vi "欣然动力数据采集系统.vi"() -> ()   [LabVIEW 2020]
uses:
  <vilib>/Utility/error.llb/DialogType.ctl
  <userlib>/ArtDAQ/_SubVI/ArtDAQ_CreateAIVoltageChan.vi
  <userlib>/ArtDAQ/_SubVI/ArtDAQ_CfgSampClkTiming.vi
  <userlib>/ArtDAQ/_SubVI/ArtDAQ_Read Analog DBL NChan NSamp.vi
  <vilib>/express/express analysis/Spectral/Block/exnSpectralBlock spectral measurements RMS poly.vi
  <vilib>/express/express analysis/Spectral/Block/exnSpectralBlock spectral measurements RMS WFM.vi
  <userlib>/ArtDAQ/_SubVI/ArtDAQ_CreateCIFreqChan.vi
  <userlib>/ArtDAQ/_SubVI/ArtDAQ_CfgImplicitTiming.vi
  <userlib>/ArtDAQ/_SubVI/ArtDAQ_Read Counter DBL NSamp.vi
  <vilib>/express/express analysis/Spectral/XNode/ExpressSpectralMeasurementsBlockNode.xnode
panel:
  out "排温2raw":dbl
  out "排温1raw":dbl format="%#.1f"
  out "推力raw":dbl caption="推力" format="%#.1f"
  in  "?":enum32{"通道及记录设置", "参数显示", "振动显示"}(tab)
  in  "流量通道":string="Dev1/ctr1"
  in  "震动通道3":string="Dev1/ai3"
  in  "震动通道2":string="Dev1/ai2"
  in  "震动通道1":string="Dev1/ai1"
  in  "排温通道2":string="Dev1/ai13"
  in  "排温通道1":string="Dev1/ai9"
  in  "推力通道":string="Dev1/ai0"
  in  "大气温度通道":string="Dev1/ai12"
  in  "大气压力通道":string="Dev1/ai11"
  in  "Filename":path=path "vibration.tdms" caption="振动参数"
  in  "记录频率":dbl=1.0
  in  "文件名":path=path "Engine_data.lvm" caption="发动机运行参数"
  in  "排温1超限报警值":dbl=800.0
  in  "排温2超限报警值":dbl=800.0
  in  "推力偏移校正":dbl
  in  "转速通道":string="Dev1/ctr0"
  in  "新建":bool
  in  "开始/暂停":bool
  out "?":dbl format="%#.0f"
  out "排温 2":dbl(knob) scale=0.0..1200.0
  out "?":dbl format="%#.0f"
  out "排温1":dbl(knob) scale=0.0..1200.0
  out "?":dbl format="%#.1f"
  out "推力":dbl(knob) scale=0.0..80.0
  out "?":dbl format="%#.1f"
  out "流量":dbl(knob) scale=0.0..3000.0
  out "?":dbl format="%#.0f"
  out "转速":dbl(knob) scale=0.0..100000.0 scale format="%#_3p"
  out "记录中 2":bool caption="记录中"
  out "发动机运行参数":dynamicdata(graph)=[{"t0"=timestamp(3721086911.630264 s since 1904-01-01), "dt"=0.1, "Y"=[0.0], "attributes"=variant("NI_ChannelName"=variant(string "滤波"))}, {"t0"=timestamp(3721086911.630264 s since 1904-01-01), "dt"=0.1, "Y"=[0.0], "attributes"=variant("NI_ChannelName"=variant(string "滤波"))}, {"t0"=timestamp(3721086911.630264 s since 1904-01-01), "dt"=0.1, "Y"=[-174.99999999999991], "attributes"=variant("NI_ChannelName"=variant(string "滤波"))}, {"t0"=timestamp(3721086911.630264 s since 1904-01-01), "dt"=0.1, "Y"=[0.0], "attributes"=variant("NI_ChannelName"=variant(string "滤波"))}, {"t0"=timestamp(3721086911.630264 s since 1904-01-01), "dt"=0.1, "Y"=[0.0], "attributes"=variant("NI_ChannelName"=variant(string "滤波"))}]
  out "大气压力":dbl format="%#.1f"
  out "机箱温度":dbl format="%#.1g"
  out "超温警报":bool
  in  "校零":bool
  in  "采样率":dbl=200000.0
  out "实际采样点数":dbl=30000.0
  in  "每循环采样数":i32=100000
  out "波形图 2":cluster{"f0":dbl, "df":dbl, "magnitude":dbl[]}(graph)
  in  "开始/暂停 2":bool
  in  "新建 2":bool
  out "波形图 3":cluster{"f0":dbl, "df":dbl, "magnitude":dbl[]}(graph) caption="波形图 2"
  out "波形图 4":cluster{"f0":dbl, "df":dbl, "magnitude":dbl[]}(graph) caption="波形图 2"
  out "加速度":waveform(dbl)[](graph)
  out "转速":dbl format="%#.0f"
  out "燃油流量":dbl caption="流量" format="%#.1f"
  # "参数记录设置"
  # "通道设置"
  # "记录频率"
  # "HZ"
  # "报警参数设置"
  # "参数校正"
  # "微型试车台数采系统 V1.1"
  # "欣然动力"
  # "kPa"
  # "r/min"
  # "ml/min"
  # "kgf"
  # "℃"
  # "℃"
  # "℃"
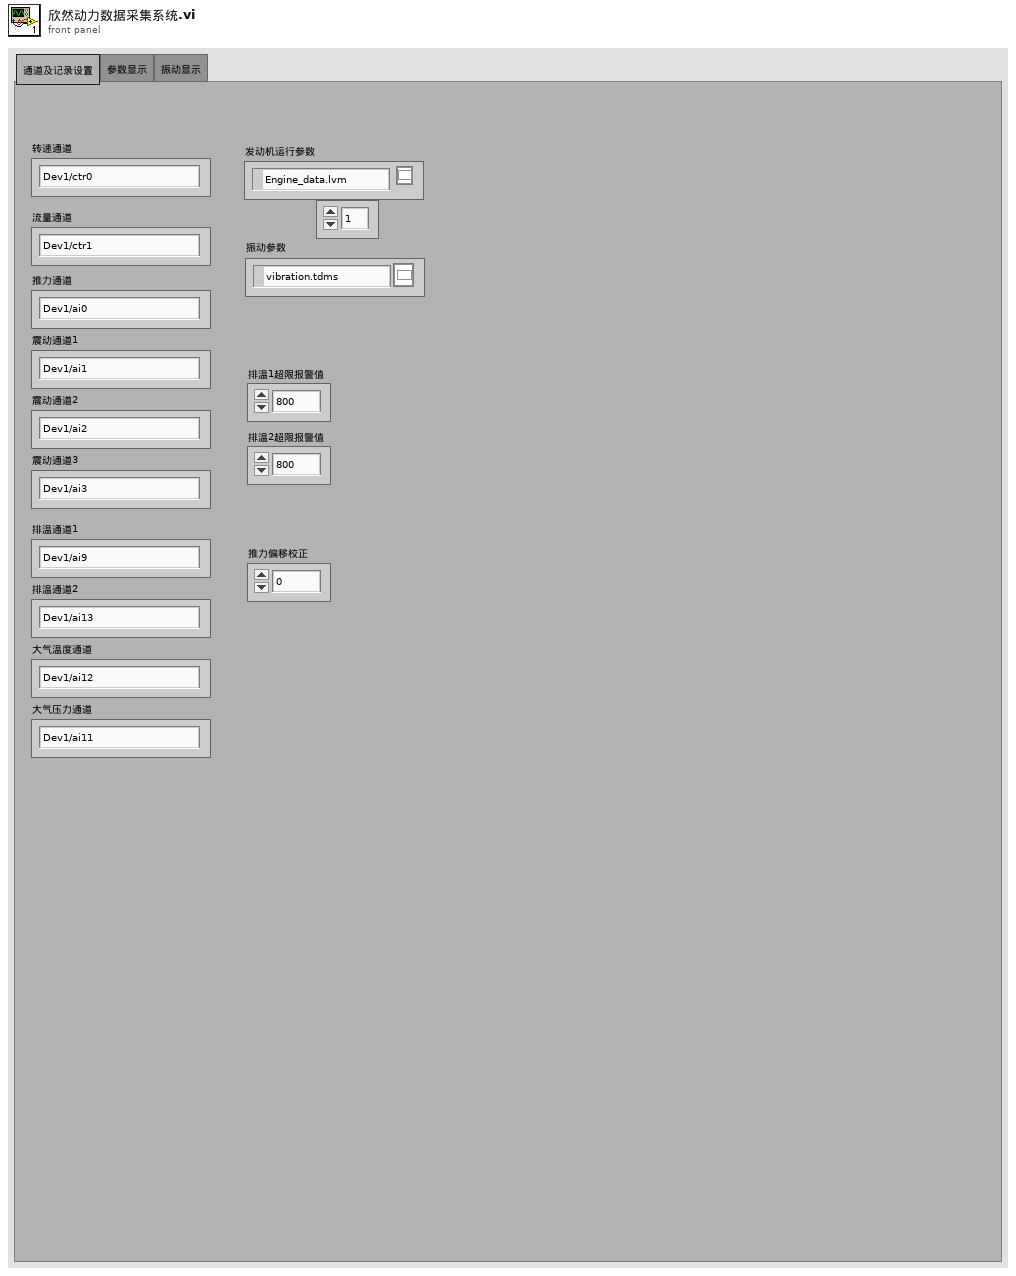
[diagram p1: front panel]
types:
  T1 = typedef "DialogType.ctl" = u16
  T2 = cluster{"averaging mode":u16, "weighting mode":u16, "number of averages":u32}
  T3 = cluster{"dB On (F)":bool, "unwrap phase (F)":bool, "convert to degree (F)":bool}
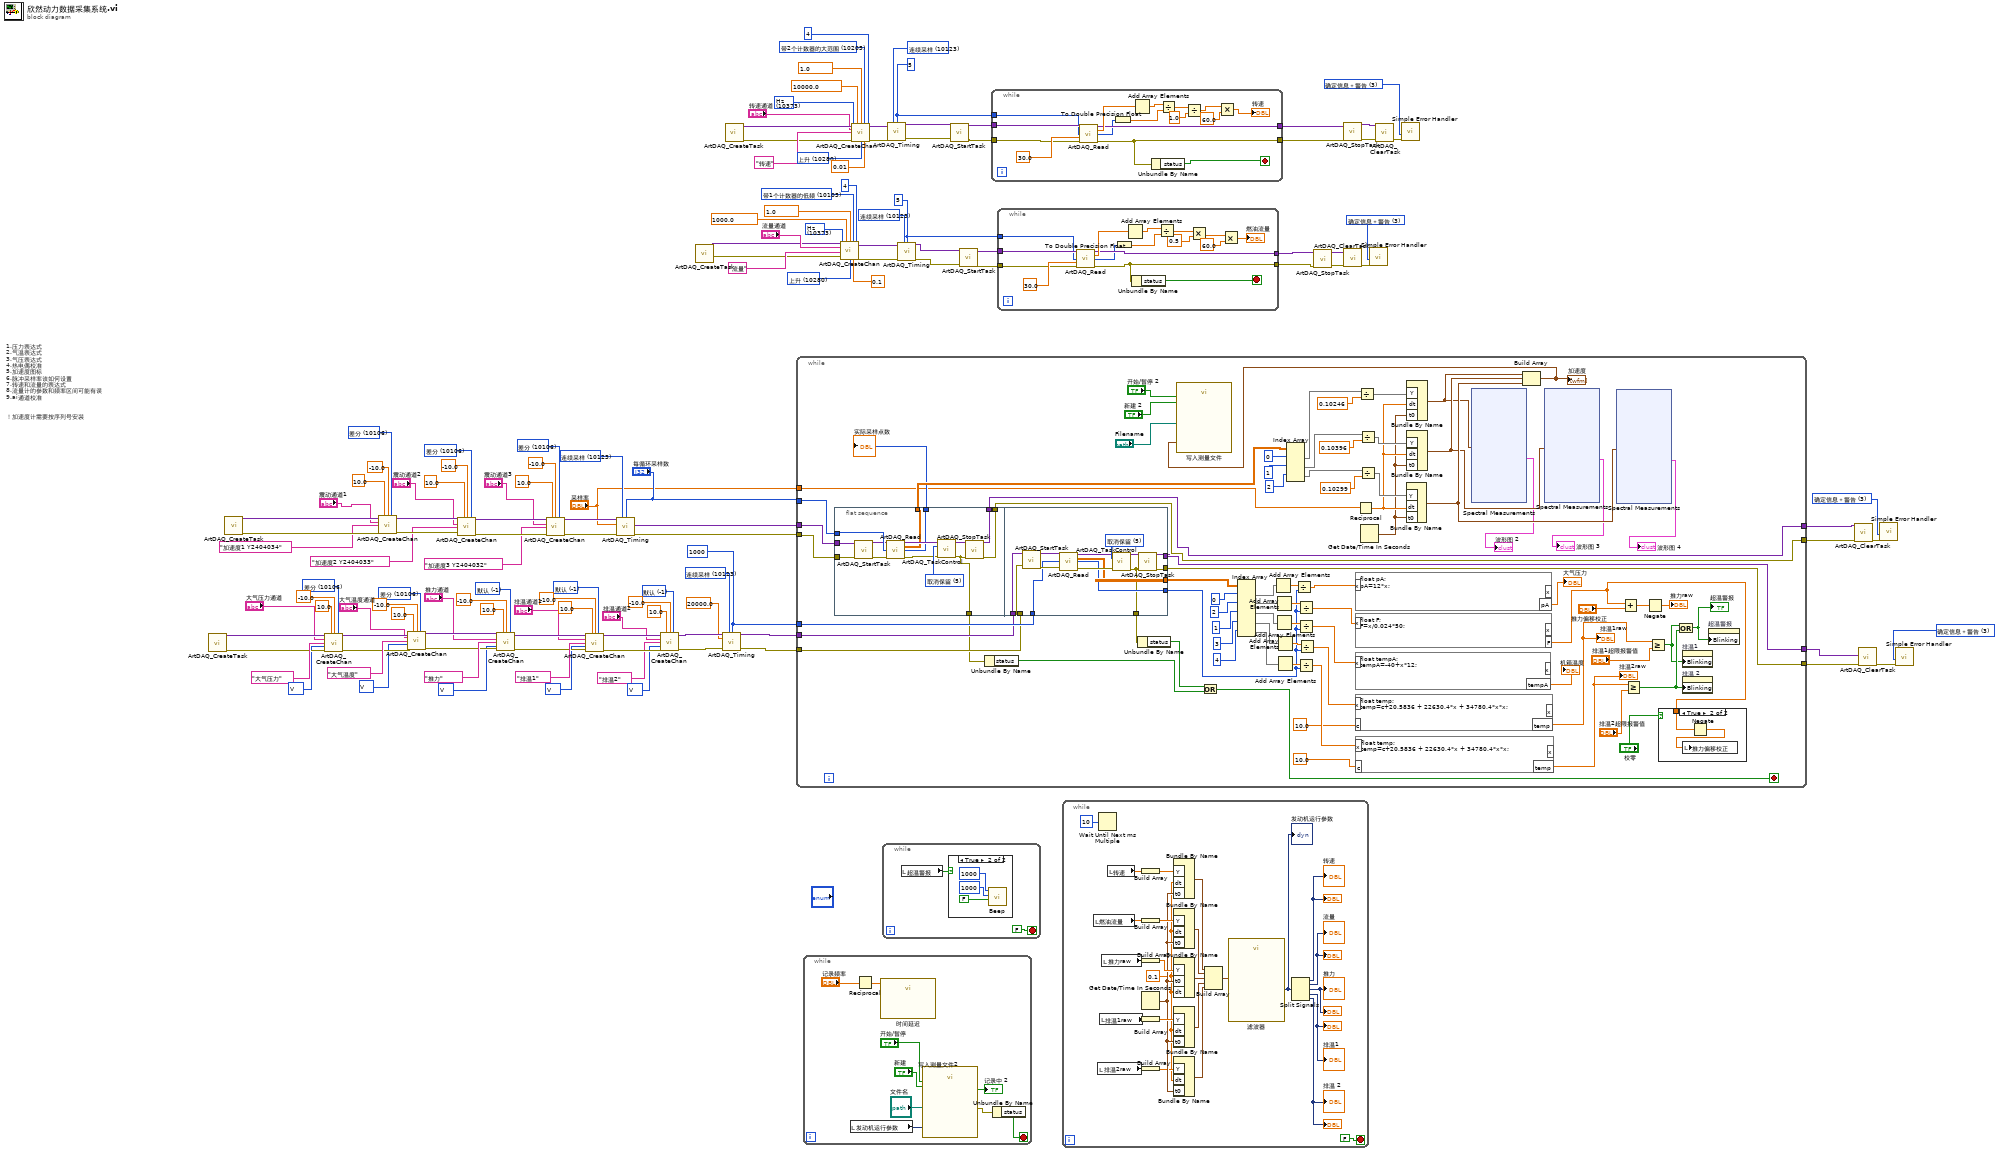
[diagram p0: block diagram]
diagram:
  w6 = 5 ("每通道点数")
  w39 = 10280 items=["上升"=10280, "下降"=10171] ("开始边沿")
  w40 = 10105 items=["带1个计数器的低频"=10105, "带2个计数器的高频"=10157, "带2个计数器的大范围"=10205] ("测量方法")
  w41 = 10373 items=["Hz"=10373, "时钟滴答"=10304, "来自自定义换算"=10065] ("Units")
  w42 = 10123 items=["有限点采样"=10178, "连续采样"=10123] ("采样模式")
  w5 = 5 ("每通道点数")
  w50 = 10280 items=["上升"=10280, "下降"=10171] ("开始边沿")
  w51 = 10205 items=["带1个计数器的低频"=10105, "带2个计数器的高频"=10157, "带2个计数器的大范围"=10205] ("测量方法")
  w52 = 10373 items=["Hz"=10373, "时钟滴答"=10304, "来自自定义换算"=10065] ("Units")
  w53 = 10123 items=["有限点采样"=10178, "连续采样"=10123] ("采样模式")
  w59 = T1 3 items=["无对话框", "确定信息", "继续或停止信息", "确定信息＋警告", "继续/停止＋警告"] ("对话框类型（确定信息：1）")
  w69 = T1 3 items=["无对话框", "确定信息", "继续或停止信息", "确定信息＋警告", "继续/停止＋警告"] ("对话框类型（确定信息：1）")
  w70 = 10106 items=["默认"=-1, "单端"=10083, "非参考单端"=10078, "差分"=10106, "伪差分"=12529] ("接线端配置")
  w71 = 10106 items=["默认"=-1, "单端"=10083, "非参考单端"=10078, "差分"=10106, "伪差分"=12529] ("接线端配置")
  w72 = 10106 items=["默认"=-1, "单端"=10083, "非参考单端"=10078, "差分"=10106, "伪差分"=12529] ("接线端配置")
  w73 = 10348 items=["V"=10348, "来自自定义换算"=10065] ("单位")
  w74 = 10348 items=["V"=10348, "来自自定义换算"=10065] ("单位")
  w75 = 10348 items=["V"=10348, "来自自定义换算"=10065] ("单位")
  w76 = 10348 items=["V"=10348, "来自自定义换算"=10065] ("单位")
  w77 = 10348 items=["V"=10348, "来自自定义换算"=10065] ("单位")
  w81 = 10123 items=["有限点采样"=10178, "连续采样"=10123] ("采样模式")
  w96 = 10123 items=["有限点采样"=10178, "连续采样"=10123] ("采样模式")
  w108 = 10106 items=["默认"=-1, "单端"=10083, "非参考单端"=10078, "差分"=10106, "伪差分"=12529] ("接线端配置")
  w112 = 10106 items=["默认"=-1, "单端"=10083, "非参考单端"=10078, "差分"=10106, "伪差分"=12529] ("接线端配置")
  w116 = -1 items=["默认"=-1, "单端"=10083, "非参考单端"=10078, "差分"=10106, "伪差分"=12529] ("接线端配置")
  w123 = -1 items=["默认"=-1, "单端"=10083, "非参考单端"=10078, "差分"=10106, "伪差分"=12529] ("接线端配置")
  w4 = 1000 ("每通道采样数")
  w126 = -1 items=["默认"=-1, "单端"=10083, "非参考单端"=10078, "差分"=10106, "伪差分"=12529] ("接线端配置")
  w132 = T1 3 items=["无对话框", "确定信息", "继续或停止信息", "确定信息＋警告", "继续/停止+警告"] ("type of dialog (OK msg:1)")
  w133 = T1 3 items=["无对话框", "确定信息", "继续或停止信息", "确定信息＋警告", "继续/停止＋警告"] ("对话框类型（确定信息：1）")
  # "1.压力表达式\n2.气温表达式\n3.气压表达式\n4.热电偶校准\n5.加速度图标\n6.脉冲采样率该如何设置\n7.转速和流量的表达式\n8.流量计的参数和频率区间可能有误\n9.ai通道校准\n\n\n！加速度计需要按序列号安装"
  n1 = call <userlib>:"ArtDAQ_CreateTask.vi"() -> ("任务句柄"=w104:variant, "错误输出"=w100:errorcluster)  [unwired: 14 in]
  n2 = call <userlib>:"ArtDAQ_CreateTask.vi"() -> ("任务句柄"=w87:variant, "错误输出"=w86:errorcluster)  [unwired: 14 in]
  n3 = call-poly <userlib>:"ArtDAQ_CreateChan.vi"("任务句柄"=w104, "最大值"=10.0, "最小值"=-10.0, "接线端配置"=w108, "物理通道"="大气压力通道", "分配名称"="大气压力", "单位"=w75, "错误输入"=w100) -> ("任务句柄"=w103:variant, "错误输出"=w99:errorcluster)  [unwired: 6 in]
  n4 = call-poly <userlib>:"ArtDAQ_CreateChan.vi"("任务句柄"=w87, "最大值"=10.0, "最小值"=-10.0, "接线端配置"=w70, "物理通道"="震动通道1", "分配名称"="加速度1 Y2404034", "错误输入"=w86) -> ("任务句柄"=w89:variant, "错误输出"=w85:errorcluster)  [unwired: 7 in]
  n5 = call-poly <userlib>:"ArtDAQ_CreateChan.vi"("任务句柄"=w103, "最大值"=10.0, "最小值"=-10.0, "接线端配置"=w112, "物理通道"="大气温度通道", "分配名称"="大气温度", "单位"=w76, "错误输入"=w99) -> ("任务句柄"=w102:variant, "错误输出"=w98:errorcluster)  [unwired: 6 in]
  n6 = call-poly <userlib>:"ArtDAQ_CreateChan.vi"("任务句柄"=w89, "最大值"=10.0, "最小值"=-10.0, "接线端配置"=w71, "物理通道"="震动通道2", "分配名称"="加速度2 Y2404033", "错误输入"=w85) -> ("任务句柄"=w88:variant, "错误输出"=w84:errorcluster)  [unwired: 7 in]
  n7 = call-poly <userlib>:"ArtDAQ_CreateChan.vi"("任务句柄"=w102, "最大值"=10.0, "最小值"=-10.0, "接线端配置"=w116, "物理通道"="推力通道", "分配名称"="推力", "单位"=w77, "错误输入"=w98) -> ("任务句柄"=w101:variant, "错误输出"=w97:errorcluster)  [unwired: 6 in]
  n8 = call-poly <userlib>:"ArtDAQ_CreateChan.vi"("任务句柄"=w88, "最大值"=10.0, "最小值"=-10.0, "接线端配置"=w72, "物理通道"="震动通道3", "分配名称"="加速度3 Y2404032", "错误输入"=w84) -> ("任务句柄"=w83:variant, "错误输出"=w82:errorcluster)  [unwired: 7 in]
  n9 = call-poly <userlib>:"ArtDAQ_CreateChan.vi"("任务句柄"=w101, "最大值"=10.0, "最小值"=-10.0, "接线端配置"=w123, "物理通道"="排温通道1", "分配名称"="排温1", "单位"=w74, "错误输入"=w97) -> ("任务句柄"=w120:variant, "错误输出"=w119:errorcluster)  [unwired: 6 in]
  n10 = call-poly <userlib>:"ArtDAQ_Timing.vi"("任务句柄"=w83, "采样模式"=w81, "每通道采样数"="每循环采样数", "采样率"="采样率", "错误输入"=w82) -> ("任务句柄"=w28:variant, "错误输出"=w27:errorcluster)  [unwired: 9 in]
  n11 = call-poly <userlib>:"ArtDAQ_CreateChan.vi"("任务句柄"=w120, "最大值"=10.0, "最小值"=-10.0, "接线端配置"=w126, "物理通道"="排温通道2", "分配名称"="排温2", "单位"=w73, "错误输入"=w119) -> ("任务句柄"=w129:variant, "错误输出"=w128:errorcluster)  [unwired: 6 in]
  n12 = call <userlib>:"ArtDAQ_CreateTask.vi"() -> ("任务句柄"=w31:variant, "错误输出"=w30:errorcluster)  [unwired: 14 in]
  n13 = call-poly <userlib>:"ArtDAQ_Timing.vi"("任务句柄"=w129, "采样模式"=w96, "每通道采样数"=w4, "采样率"=20000.0, "错误输入"=w128) -> ("任务句柄"=w24:variant, "错误输出"=w23:errorcluster)  [unwired: 9 in]
  n14 = call <userlib>:"ArtDAQ_CreateTask.vi"() -> ("任务句柄"=w35:variant, "错误输出"=w36:errorcluster)  [unwired: 14 in]
  n15 = while {
    tunnel: "每循环采样数" -> [w213]
    tunnel: w4 -> [w212]
    tunnel: w28 -> [w211]
    tunnel: w27 -> [w208]
    tunnel: [w141] -> w26
    tunnel: [w142] -> w25
    tunnel: w24 -> [w210]
    tunnel: w23 -> [w209]
    tunnel: [w140] -> w3
    tunnel: [w139] -> w2
    tunnel: "采样率" -> [w134]
    stop <- w136 stop-if-true
    n16 = flat-sequence {
      tunnel: w213 -> [w256]
      tunnel: w211 -> [w255]
      tunnel: w208 -> [w254]
      tunnel: [w250] -> w140
      tunnel: [w249] -> w139
      tunnel: [w248] -> w137
      tunnel: [w247] -> w138
      tunnel: [w246] -> w184
      tunnel: w212 -> [w263]
      tunnel: [w271] -> w141
      tunnel: [w264] -> w142
      tunnel: w210 -> [w270]
      tunnel: w209 -> [w269]
      tunnel: [w262] -> w146
      tunnel: [w261] -> w152
      tunnel: [w260] -> w143
      frame #0 {
        w259 = 5 items=["开始", "停止", "验证", "提交", "保留", "取消保留", "中止"] ("动作")
        n17 = call <userlib>:"ArtDAQ_StartTask.vi"("任务句柄"=w255, "错误输入"=w254) -> ("任务句柄"=w253:variant, "错误输出"=w252:errorcluster)  [unwired: 12 in]
        n18 = call-poly <userlib>:"ArtDAQ_Read.vi"("任务句柄"=w253, "每通道采样数"=w256, "错误输入"=w252) -> ("任务句柄"=w258:variant, "数据"=w247:dbl[][], "实际读取点数"=w248:i32, "错误输出"=w257:errorcluster)  [unwired: 9 in]
        n19 = call <userlib>:"ArtDAQ_TaskControl.vi"("任务句柄"=w258, "动作"=w259, "错误输入"=w257) -> ("任务句柄"=w251:variant, "错误输出"=w246:errorcluster)  [unwired: 11 in]
        n20 = call <userlib>:"ArtDAQ_StopTask.vi"("任务句柄"=w251, "错误输入"=w246) -> ("任务句柄"=w250:variant, "错误输出"=w249:errorcluster)  [unwired: 12 in]
      }
      frame #1 {
        w273 = 5 items=["开始", "停止", "验证", "提交", "保留", "取消保留", "中止"] ("动作")
        n21 = call <userlib>:"ArtDAQ_StartTask.vi"("任务句柄"=w270, "错误输入"=w269) -> ("任务句柄"=w268:variant, "错误输出"=w267:errorcluster)  [unwired: 12 in]
        n22 = call-poly <userlib>:"ArtDAQ_Read.vi"("任务句柄"=w268, "每通道采样数"=w263, "错误输入"=w267) -> ("任务句柄"=w266:variant, "数据"=w261:dbl[][], "实际读取点数"=w262:i32, "错误输出"=w265:errorcluster)  [unwired: 9 in]
        n23 = call <userlib>:"ArtDAQ_TaskControl.vi"("任务句柄"=w266, "动作"=w273, "错误输入"=w265) -> ("任务句柄"=w272:variant, "错误输出"=w260:errorcluster)  [unwired: 11 in]
        n24 = call <userlib>:"ArtDAQ_StopTask.vi"("任务句柄"=w272, "错误输入"=w260) -> ("任务句柄"=w271:variant, "错误输出"=w264:errorcluster)  [unwired: 12 in]
      }
    }
    n25 = Unbundle By Name(w184) -> ("status"=w183:bool)
    n26 = Unbundle By Name(w143) -> ("status"=w144:bool)
    n27 = Or(x=w144, y=w183) -> (x .or. y?=w136:bool)
    n28 = Index Array(array=w152, index (row) #1=0 ("index (row)"), index (row) #2=2 ("index (row)"), index (row) #3=1 ("index (row)"), index (row) #4=3 ("index (row)"), index (row) #5=4 ("index (row)")) -> (element #1=w155:dbl[], element #2=w160:dbl[], element #3=w161:dbl[], element #4=w162:dbl[], element #5=w163:dbl[])  [unwired: 5 in]
    n29 = Add Array Elements(numeric array=w155) -> (sum=w154:dbl)
    n30 = Add Array Elements(numeric array=w160) -> (sum=w156:dbl)
    n31 = Add Array Elements(numeric array=w161) -> (sum=w157:dbl)
    n32 = Add Array Elements(numeric array=w162) -> (sum=w158:dbl)
    n33 = Add Array Elements(numeric array=w163) -> (sum=w159:dbl)
    n34 = Index Array(array=w138, index (row) #1=0 ("index (row)"), index (row) #2=1 ("index (row)"), index (row) #3=2 ("index (row)")) -> (element #1=w199:dbl[], element #2=w202:dbl[], element #3=w203:dbl[])  [unwired: 3 in]
    n35 = Divide(x=w154, y=w146) -> (x/y=w164:dbl)
    n36 = Divide(x=w156, y=w146) -> (x/y=w165:dbl)
    n37 = Divide(x=w157, y=w146) -> (x/y=w166:dbl)
    n38 = Divide(x=w159, y=w146) -> (x/y=w168:dbl)
    n39 = Divide(x=w158, y=w146) -> (x/y=w167:dbl)
    n40 = formula code="float pA;\npA=12*x;"("x"=w164) -> ("pA"=→"大气压力":dbl)  [unwired: 1 out]
    n41 = formula code="float F;\nF=x/0.024*50;"("x"=w165) -> ("F"=w179:dbl)  [unwired: 1 out]
    n42 = formula code="float tempA;\ntempA=-40+x*12;"("x"=w166) -> ("tempA"=→"机箱温度":dbl)  [unwired: 1 out]
    n43 = formula code="float temp;\ntemp=c+20.5836 + 22630.4*x + 34780.4*x*x;"("x"=w167, "c"=10.0 ("input variable")) -> ("temp"=w177:dbl)  [unwired: 1 out]
    "排温1raw" <- w177
    n44 = formula code="float temp;\ntemp=c+20.5836 + 22630.4*x + 34780.4*x*x;"("x"=w168, "c"=10.0 ("input variable")) -> ("temp"=w180:dbl)  [unwired: 1 out]
    "排温2raw" <- w180
    n45 = Reciprocal(x=w134) -> (1/x=w192:dbl)
    n46 = Divide(x=w199, y=0.10246 ("最小值")) -> (x/y=w200:dbl[])
    n47 = Divide(x=w202, y=0.10396 ("最小值")) -> (x/y=w201:dbl[])
    n48 = Divide(x=w203, y=0.10299 ("最小值")) -> (x/y=w204:dbl[])
    n49 = Get Date/Time In Seconds() -> (seconds since 1Jan1904=w191:timestamp)
    n50 = Bundle By Name("Y"=w204, "dt"=w192, "t0"=w191) -> (w198:waveform(dbl))  [unwired: 1 in]
    n51 = Bundle By Name("Y"=w200, "dt"=w192, "t0"=w191) -> (w196:waveform(dbl))  [unwired: 1 in]
    n52 = Bundle By Name("Y"=w201, "dt"=w192, "t0"=w191) -> (w197:waveform(dbl))  [unwired: 1 in]
    n53 = xnode "Spectral Measurements"("Signals"=w196) -> ("FFT - (RMS)"=→"波形图 2":cluster{"f0":dbl, "df":dbl, "magnitude":dbl[]})  [unwired: 1 in, 2 out]
    n54 = Build Array(w196, w197, w198) -> (w135:waveform(dbl)[])
    "加速度" <- w135
    n55 = call "写入测量文件"("Signals"=w135, "Enable"="开始/暂停 2", "new_file"="新建 2", "Filename"="Filename") -> ()  [unwired: 13 in, 3 out]
    n56 = xnode "Spectral Measurements"("Signals"=w197) -> ("FFT - (RMS)"=→"波形图 3":cluster{"f0":dbl, "df":dbl, "magnitude":dbl[]})  [unwired: 1 in, 2 out]
    n57 = xnode "Spectral Measurements"("Signals"=w198) -> ("FFT - (RMS)"=→"波形图 4":cluster{"f0":dbl, "df":dbl, "magnitude":dbl[]})  [unwired: 1 in, 2 out]
    n58 = Add(x=w179, y="推力偏移校正") -> (x+y=w170:dbl)
    n59 = Greater Or Equal?(x=w180, y="排温2超限报警值") -> (x >= y?=w182:bool)
    n60 = Negate(x=w170) -> (-x=→"推力raw":dbl)
    n61 = Greater Or Equal?(x=w177, y="排温1超限报警值") -> (x >= y?=w181:bool)
    n62 = case shown="True" "校零" {
      tunnel: w179 -> [_ w215]
      frame False {
      }
      frame True {
        n63 = Negate(x=w215) -> (-x=w214:dbl)
        n64 = local write "推力偏移校正"(w214) -> ()
      }
    }
    n65 = Or(x=w181, y=w182) -> (x .or. y?=w173:bool)
    "超温警报" <- w173
    n66 = property on="排温1" class="Knob (strict)"("Blinking"=w181) -> ()  [unwired: 2 in, 2 out]
    n67 = property on="排温 2" class="Knob (strict)"("Blinking"=w182) -> ()  [unwired: 2 in, 2 out]
    n68 = property on="超温警报" class="Bool (strict)"("Blinking"=w173) -> ()  [unwired: 2 in, 2 out]
    "实际采样点数" <- w137
  }
  n69 = while {
    stop <- w274 stop-if-true
    n70 = local read "发动机运行参数"() -> (w280:dynamicdata)
    n71 = Reciprocal(x="记录频率") -> (1/x=w276:dbl)
    n72 = call "时间延迟"("Delay Time (s)"=w276) -> ()  [unwired: 10 in, 1 out]
    n73 = call "写入测量文件2"("Signals"=w280, "Enable"="开始/暂停", "new_file"="新建", "Filename"="文件名") -> ("Saving Data"=→"记录中 2":bool, "error out"=w275:errorcluster)  [unwired: 13 in, 1 out]
    n74 = Unbundle By Name(w275) -> ("status"=w274:bool)
  }
  n75 = call-poly <userlib>:"ArtDAQ_CreateChan.vi"("任务句柄"=w31, "最大值"=1000.0, "最小值"=1.0, "测量方法"=w40, "计数器"="流量通道", "除数"=u32 4, "分配名称"="流量", "单位"=w41, "错误输入"=w30, "开始边沿"=w39, "测量时间"=0.1) -> ("任务句柄"=w44:variant, "错误输出"=w43:errorcluster)  [unwired: 3 in]
  n76 = call-poly <userlib>:"ArtDAQ_CreateChan.vi"("任务句柄"=w35, "最大值"=10000.0, "最小值"=1.0, "测量方法"=w51, "计数器"="转速通道", "除数"=u32 4, "分配名称"="转速", "单位"=w52, "错误输入"=w36, "开始边沿"=w50, "测量时间"=0.01) -> ("任务句柄"=w55:variant, "错误输出"=w54:errorcluster)  [unwired: 3 in]
  n77 = while {
    stop <- FALSE stop-if-true
    n78 = local read "超温警报"() -> (w284:bool)
    n79 = case shown="True" w284 {
      frame False {
      }
      frame True {
        n80 = call <vilib>:"Beep.vi"("use system alert? (T)"=FALSE, "duration (msec)"=u32 1000, "frequency (Hz)"=u32 1000) -> ()  [unwired: 9 in]
      }
    }
  }
  n81 = call-poly <userlib>:"ArtDAQ_Timing.vi"("任务句柄"=w55, "采样模式"=w53, "每通道采样数"=w5, "错误输入"=w54) -> ("任务句柄"=w16:variant, "错误输出"=w15:errorcluster)  [unwired: 10 in]
  n82 = call-poly <userlib>:"ArtDAQ_Timing.vi"("任务句柄"=w44, "采样模式"=w42, "每通道采样数"=w6, "错误输入"=w43) -> ("任务句柄"=w8:variant, "错误输出"=w7:errorcluster)  [unwired: 10 in]
  n83 = call <userlib>:"ArtDAQ_StartTask.vi"("任务句柄"=w16, "错误输入"=w15) -> ("任务句柄"=w17:variant, "错误输出"=w18:errorcluster)  [unwired: 12 in]
  n84 = call <userlib>:"ArtDAQ_StartTask.vi"("任务句柄"=w8, "错误输入"=w7) -> ("任务句柄"=w10:variant, "错误输出"=w9:errorcluster)  [unwired: 12 in]
  n85 = while {
    tunnel: [w297] -> w20
    tunnel: [w296] -> w19
    tunnel: w18 -> [w295]
    tunnel: w17 -> [w294]
    tunnel: w5 -> [w292]
    stop <- w293 stop-if-true
    n86 = call-poly <userlib>:"ArtDAQ_Read.vi"("任务句柄"=w294, "每通道采样数"=w292, "超时s"=30.0, "错误输入"=w295) -> ("任务句柄"=w297:variant, "数据"=w298:dbl[], "实际读取点数"=w291:i32, "错误输出"=w296:errorcluster)  [unwired: 8 in]
    n87 = To Double Precision Float(number=w291) -> (double precision float=w300:dbl)
    n88 = Add Array Elements(numeric array=w298) -> (sum=w301:dbl)
    n89 = Unbundle By Name(w296) -> ("status"=w293:bool)
    n90 = Divide(x=w301, y=w300) -> (x/y=w302:dbl)
    n91 = Divide(x=w302, y=1.0) -> (x/y=w289:dbl)
    n92 = Multiply(x=w289, y=60.0) -> (x*y=→"转速":dbl)
  }
  n93 = while {
    tunnel: [w312] -> w14
    tunnel: [w309] -> w13
    tunnel: w10 -> [w311]
    tunnel: w9 -> [w310]
    tunnel: w6 -> [w308]
    stop <- w313 stop-if-true
    n94 = call-poly <userlib>:"ArtDAQ_Read.vi"("任务句柄"=w311, "每通道采样数"=w308, "超时s"=30.0, "错误输入"=w310) -> ("任务句柄"=w312:variant, "数据"=w314:dbl[], "实际读取点数"=w307:i32, "错误输出"=w309:errorcluster)  [unwired: 8 in]
    n95 = To Double Precision Float(number=w307) -> (double precision float=w317:dbl)
    n96 = Add Array Elements(numeric array=w314) -> (sum=w316:dbl)
    n97 = Unbundle By Name(w309) -> ("status"=w313:bool)
    n98 = Divide(x=w316, y=w317) -> (x/y=w318:dbl)
    n99 = Multiply(x=w318, y=0.5) -> (x*y=w305:dbl)
    n100 = Multiply(x=w305, y=60.0) -> (x*y=→"燃油流量":dbl)
  }
  n101 = while {
    stop <- FALSE stop-if-true
    w322 = 0.1 ("dt")
    n102 = local read "燃油流量"() -> (w344:dbl)
    n103 = local read "排温2raw"() -> (w324:dbl)
    n104 = Wait Until Next ms Multiple(millisecond multiple=u32 10 ("毫秒倍数")) -> ()  [unwired: 1 out]
    n105 = local read "排温1raw"() -> (w339:dbl)
    n106 = local read "推力raw"() -> (w341:dbl)
    n107 = local read "转速"() -> (w342:dbl)
    n108 = Build Array(w342) -> (w336:dbl[])
    n109 = Build Array(w344) -> (w343:dbl[])
    n110 = Build Array(w341) -> (w340:dbl[])
    n111 = Get Date/Time In Seconds() -> (seconds since 1Jan1904=w325:timestamp)
    n112 = Build Array(w339) -> (w338:dbl[])
    n113 = Build Array(w324) -> (w323:dbl[])
    n114 = Bundle By Name("Y"=w336, "dt"=w322, "t0"=w325) -> (w331:waveform(dbl))  [unwired: 1 in]
    n115 = Bundle By Name("Y"=w343, "dt"=w322, "t0"=w325) -> (w333:waveform(dbl))  [unwired: 1 in]
    n116 = Bundle By Name("Y"=w340, "t0"=w325, "dt"=w322) -> (w337:waveform(dbl))  [unwired: 1 in]
    n117 = Bundle By Name("Y"=w338, "dt"=w322, "t0"=w325) -> (w335:waveform(dbl))  [unwired: 1 in]
    n118 = Bundle By Name("Y"=w323, "dt"=w322, "t0"=w325) -> (w321:waveform(dbl))  [unwired: 1 in]
    n119 = Build Array(w331, w333, w337, w335, w321) -> (w332:waveform(dbl)[])
    n120 = call "滤波器"("Signal"=w332) -> ("Filtered Signal"=w330:dynamicdata)  [unwired: 9 in, 1 out]
    "发动机运行参数" <- w330
    n121 = Split Signals(w330) -> (→"转速" →"?":dynamicdata, →"流量" →"?":dynamicdata, →"推力" →"?":dynamicdata, →"排温1" →"?":dynamicdata, →"排温 2" →"?":dynamicdata)  [unwired: 5 in]
  }
  n122 = call <userlib>:"ArtDAQ_StopTask.vi"("任务句柄"=w14, "错误输入"=w13) -> ("任务句柄"=w12:variant, "错误输出"=w11:errorcluster)  [unwired: 12 in]
  n123 = call <userlib>:"ArtDAQ_StopTask.vi"("任务句柄"=w20, "错误输入"=w19) -> ("任务句柄"=w22:variant, "错误输出"=w21:errorcluster)  [unwired: 12 in]
  n124 = call <userlib>:"ArtDAQ_ClearTask.vi"("任务句柄"=w12, "错误输入"=w11) -> ("错误输出"=w68:errorcluster)  [unwired: 13 in]
  n125 = call <vilib>:"Simple Error Handler.vi"("type of dialog (OK msg:1)"=w69, "error in (no error)"=w68) -> ()  [unwired: 3 in, 5 out]
  n126 = call <userlib>:"ArtDAQ_ClearTask.vi"("任务句柄"=w22, "错误输入"=w21) -> ("错误输出"=w58:errorcluster)  [unwired: 13 in]
  n127 = call <vilib>:"Simple Error Handler.vi"("type of dialog (OK msg:1)"=w59, "error in (no error)"=w58) -> ()  [unwired: 3 in, 5 out]
  n128 = call <userlib>:"ArtDAQ_ClearTask.vi"("任务句柄"=w3, "错误输入"=w2) -> ("错误输出"=w130:errorcluster)  [unwired: 13 in]
  n129 = call <userlib>:"ArtDAQ_ClearTask.vi"("任务句柄"=w26, "错误输入"=w25) -> ("错误输出"=w131:errorcluster)  [unwired: 13 in]
  n130 = call <vilib>:"Simple Error Handler.vi"("type of dialog (OK msg:1)"=w133, "error in (no error)"=w130) -> ()  [unwired: 3 in, 5 out]
  n131 = call <vilib>:"Simple Error Handler.vi"("type of dialog (OK msg:1)"=w132, "error in (no error)"=w131) -> ()  [unwired: 3 in, 5 out]
